vi "Adjust Dashboard Window.vi"(6 "Sizing Refnums":T1, 9 "Size Constraints":cluster{"min tab width":i32, "w/h":dbl}, 10 "VI":refnum<vi>, 11 "WIn Mode":refnum<notifier>) -> ()   [LabVIEW 2015]
uses:
  <vilib>/Utility/miscctls.llb/LVRectTypeDef.ctl
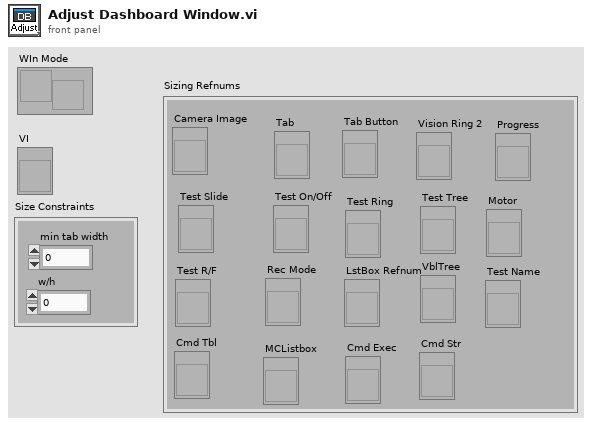
[diagram p1: front panel]
types:
  T1 = cluster{"Camera Image":refnum<vi>, "Tab":refnum<vi>, "Tab Button":refnum<vi>, "Vision Ring 2":refnum<vi>, "Rec Mode":refnum<vi>, "Test Slide":refnum<vi>, "Test On/Off":refnum<vi>, "Test Ring":refnum<vi>, "Test R/F":refnum<vi>, "Test Name":refnum<vi>, "Motor":refnum<vi>, "Progress":refnum<vi>, "LstBox Refnum":refnum<vi>, "Test Tree":refnum<vi>, "VblTree":refnum<vi>, "Cmd Tbl":refnum<vi>, "MCListbox":refnum<vi>, "Cmd Exec":refnum<vi>, "Cmd Str":refnum<vi>}
  T2 = typedef "LVPointTypeDef.ctl" = cluster{"Horizontal":i16, "Vertical":i16}
  T3 = typedef "LVRectTypeDef.ctl" = cluster{"Left":i16, "Top":i16, "Right":i16, "Bottom":i16}
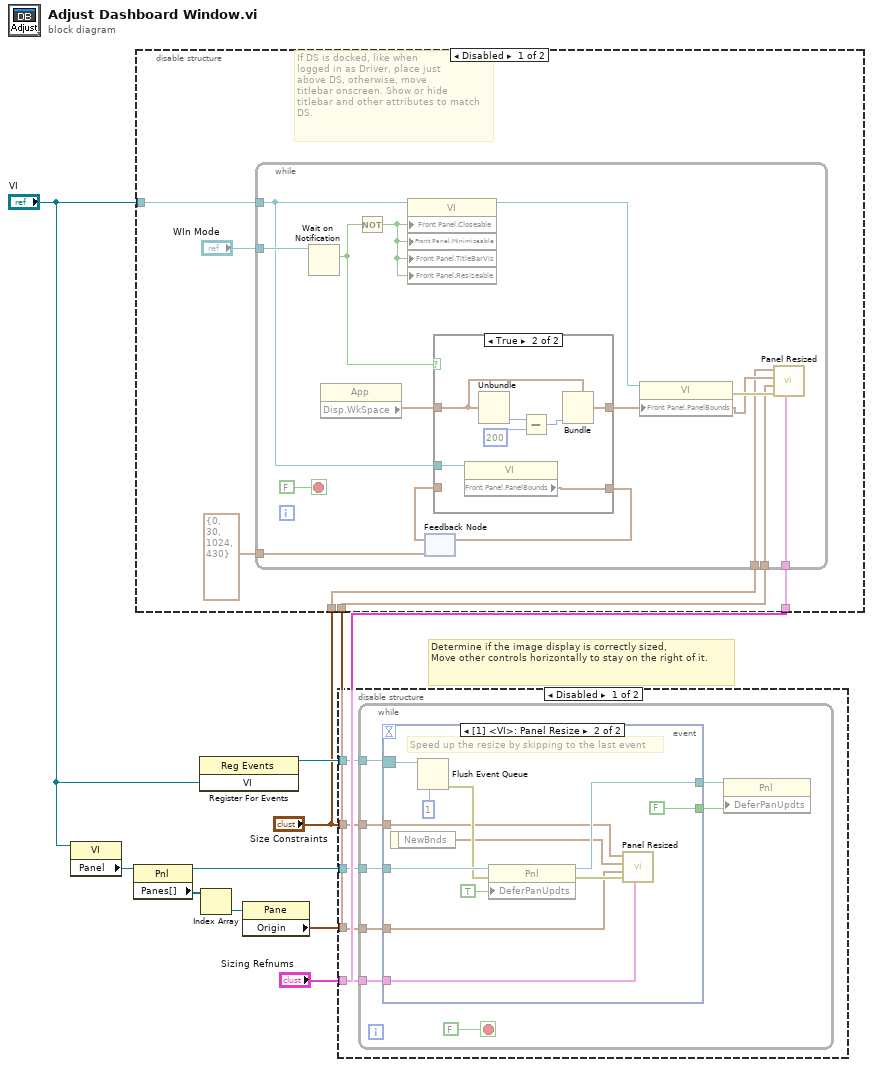
[diagram p0: block diagram]
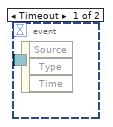
[diagram p4: hidden frame]
diagram:
  # "Determine if the image display is correctly sized,\nMove other controls horizontally to stay on the right of it."
  n1 = property class="VI"(reference="VI") -> ("Panel"=w7:refnum<vi>)  [unwired: 1 in, 2 out]
  n2 = property class="Pnl"(reference=w7) -> (reference out=w4:refnum<vi>, "Panes[]"=w6:refnum<vi>[])  [unwired: 1 in, 1 out]
  n3 = register-events("VI") -> (reference out=w9:refnum<event-registration>)  [unwired: 2 in, 1 out]
  n4 = Index Array(array=w6) -> (element=w5:refnum<vi>)  [unwired: 1 in]
  n5 = property class="Pane"(reference=w5) -> ("Origin"=w2:T2)  [unwired: 1 in, 2 out]
  n6 = disable-structure shown="Disabled" {
    disable-tunnel: "VI" -> [w14 _]
    disable-tunnel: "Sizing Refnums" -> [w13 _]
    disable-tunnel: w2 -> [w12 _]
    disable-tunnel: "Size Constraints" -> [w11 _]
    frame Disabled {
      # "If DS is docked, like when\nlogged in as Driver, place just\nabove DS, otherwise, move\ntitlebar onscreen. Show or hide\ntitlebar and other attributes to match\nDS."
      n7 = while {
        tunnel: "WIn Mode" -> [w29]
        tunnel: w14 -> [w20]
        tunnel: w13 -> [w25]
        tunnel: w12 -> [w24]
        tunnel: w11 -> [w22]
        tunnel: T3 {"Left"=0, "Top"=30, "Right"=1024, "Bottom"=430} ("Front Panel.PanelBounds") -> [w17]
        stop <- FALSE stop-if-true
        n8 = Wait on Notification(notifier=w29) -> (notification=w21:bool)  [unwired: 3 in, 3 out]
        n9 = property class="App"() -> ("Disp.WkSpace"=w28:T3)  [unwired: 2 in, 2 out]
        n10 = Not(x=w21) -> (.not. x?=w16:bool)
        n11 = property class="VI"(reference=w20, "Front Panel.Closeable"=w16, "Front Panel.Minimizeable"=w16, "Front Panel.TitleBarVis"=w16, "Front Panel.Resizeable"=w16) -> (reference out=w27:refnum<vi>)  [unwired: 1 in, 1 out]
        n12 = feedback #1(w17) -> (w18:T3)
        n13 = case shown="True" w21 {
          tunnel: w28 -> [_ w34]
          tunnel: [w31 w35] -> w23
          tunnel: w20 -> [_ w33]
          tunnel: [w31 w32] -> w19
          tunnel: w18 -> [w31 _]
          frame False {
          }
          frame True {
            n14 = property class="VI"(reference=w33) -> ("Front Panel.PanelBounds"=w32:T3)  [unwired: 1 in, 2 out]
            n15 = Unbundle(w34) -> ("Bottom"=w38:i16)  [unwired: 3 out]
            n16 = Subtract(x=w38, y=200) -> (x-y=w36:i32)
            n17 = Bundle(cluster=w34, "Bottom"=w36) -> (w35:T3)  [unwired: 3 out]
          }
        }
        n18 = feedback-in #1(w19) -> ()
        n19 = property class="VI"(reference=w27, "Front Panel.PanelBounds"=w23) -> (error out=w26:errorcluster)  [unwired: 1 in, 1 out]
        n20 = call "Panel Resized.vi"("Sizing Refnums"=w25, "error in (no error)"=w26, "Origin"=w24, "NewBnds"=w23, "Size Constraints"=w22) -> ()  [unwired: 6 in, 1 out]
      }
    }
    frame Enabled {
    }
  }
  n21 = disable-structure shown="Disabled" {
    disable-tunnel: w9 -> [w43 _]
    disable-tunnel: w4 -> [w42 _]
    disable-tunnel: "Sizing Refnums" -> [w41 _]
    disable-tunnel: w2 -> [w40 _]
    disable-tunnel: "Size Constraints" -> [w39 _]
    frame Disabled {
      n22 = while {
        tunnel: w43 -> [w50]
        tunnel: w41 -> [w49]
        tunnel: w39 -> [w48]
        tunnel: w40 -> [w47]
        tunnel: w42 -> [w46]
        stop <- FALSE stop-if-true
        n23 = event shown="[1] <VI>: Panel Resize" {
          selector: w50 -> [_ w60]
          dyn-events: _ -> [_ _]
          timeout: _ -> [_ _]
          tunnel: w49 -> [_ w52]
          tunnel: w48 -> [_ w55]
          tunnel: w47 -> [_ w53]
          tunnel: w46 -> [_ w63]
          tunnel: [_ FALSE ("Defer Panel Updates")] -> w45
          tunnel: [_ w57] -> w44
          event Timeout {
            n24 = event-data() -> ()  [unwired: 1 in, 3 out]
          }
          event Panel Resize {
            # "Speed up the resize by skipping to the last event"
            n25 = event-data() -> ("NewBnds"=w54:T3)  [unwired: 1 in]
            n26 = Flush Event Queue(0:w60, 5:1 ("keep most recent")) -> (11:w58:errorcluster)  [unwired: 4 in, 2 out]
            n27 = property class="Pnl"(reference=w63, error in=w58, "DeferPanUpdts"=TRUE ("Defer Panel Updates")) -> (reference out=w57:refnum<vi>, error out=w56:errorcluster)
            n28 = call "Panel Resized.vi"("Sizing Refnums"=w52, "error in (no error)"=w56, "Origin"=w53, "NewBnds"=w54, "Size Constraints"=w55) -> ()  [unwired: 6 in, 1 out]
          }
        }
        n29 = property class="Pnl"(reference=w44, "DeferPanUpdts"=w45) -> ()  [unwired: 1 in, 2 out]
      }
    }
    frame Enabled {
    }
  }
